vi "GOMDBTS2048 set Wavelength Range.vi"(7 "dL":dbl, 8 "error in (no error)":errorcluster, 9 "L2":dbl, 10 "L1":dbl, 11 "handle":i32) -> (0 "error out":errorcluster, 3 "function return":i32)   [LabVIEW 2015, in "GOMDBTS2048.lvlib"]
doc: "GOBTS2048DLL int __stdcall GOMDBTS2048_setWavelengthRange(int handle, double L1, double L2, double dL);"
uses:
  GOMDBTS2048.lvlib
  runtime/GOMDBTS2048.dll
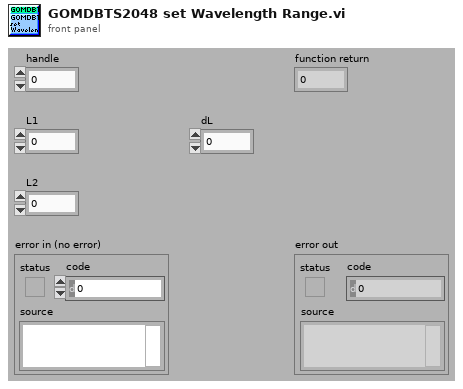
[diagram p1: front panel]
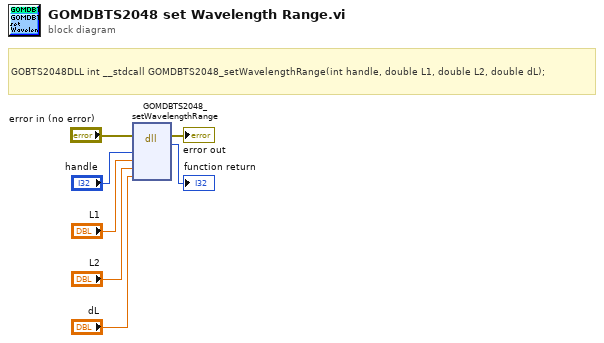
[diagram p0: block diagram]
diagram:
  # "GOBTS2048DLL int __stdcall GOMDBTS2048_setWavelengthRange(int handle, double L1, double L2, double dL);"
  n1 = dll-call lib="C:/Users/rkoch/Documents/GO_Library/runtime/GOMDBTS2048.*" fn="GOMDBTS2048_setWavelengthRange"(error in="error in (no error)", "handle"="handle", "L1"="L1", "L2"="L2", "dL"="dL") -> (error out=→"error out":errorcluster, →"function return":i32)  [unwired: 6 in, 1 out]
